vi "Set VI Icon.vi"(8 "error in (no error)":errorcluster, 10 "路径":path, 11 "VI引用句柄":refnum<vi>) -> (0 "error out":errorcluster, 1 "OK":bool, 2 "OldHandle":u32, 3 "ImageHandle":u32)   [LabVIEW 2019]
uses:
  user32.dll
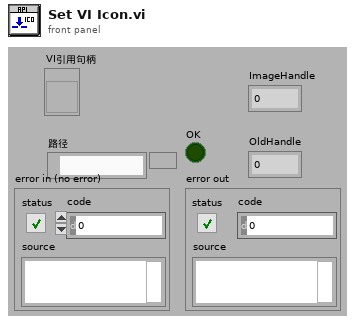
[diagram p1: front panel]
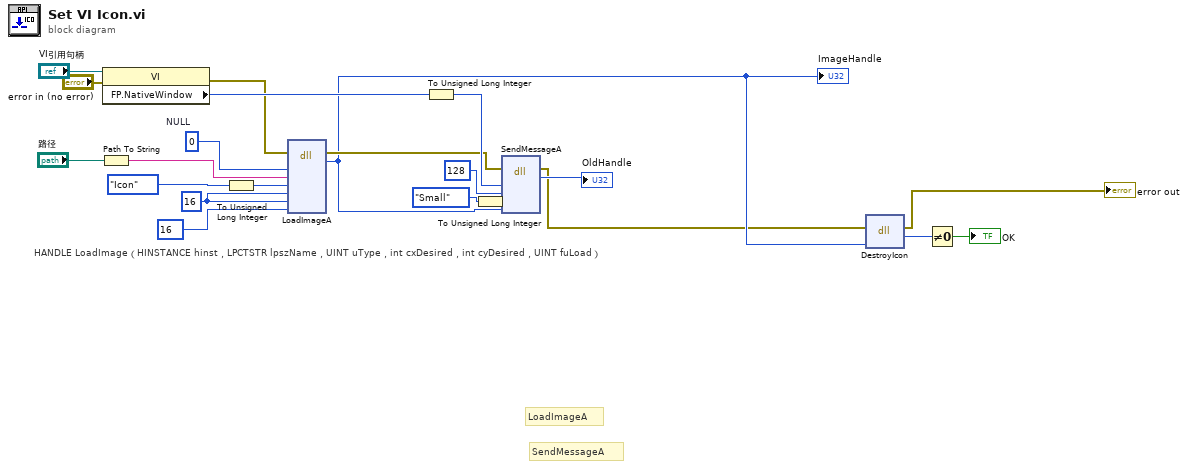
[diagram p0: block diagram]
diagram:
  w21 = u32 16 ("cxDesired")
  w22 = u32 0  # NULL
  # "SendMessageA"
  # "LoadImageA"
  # "HANDLE LoadImage（HINSTANCE hinst，LPCTSTR lpszName，UINT uType，int cxDesired，int cyDesired，UINT fuLoad）"
  n1 = Path To String(path="路径") -> (string=w19:string)
  n2 = property class="VI"(reference="VI引用句柄", error in="error in (no error)") -> (error out=w7:errorcluster, "FP.NativeWindow"=w13:u64)  [unwired: 1 out]
  n3 = To Unsigned Long Integer(number=enum32{"Bitmap", "Cursor", "Icon"}."Icon") -> (unsigned 32bit integer=w11:u32)
  n4 = dll-call lib="user32.dll" fn="LoadImageA" label="LoadImage"(error in=w7, "HINSTANCE"=w22, "LPCTSTR"=w19, "uType"=w11, "cxDesired"=w21, "cyDesired"=w21, "fuLoad"=16) -> (error out=w8:errorcluster, "ImageHandle"=w5:u32)  [unwired: 8 in, 1 out]
  "ImageHandle" <- w5
  n5 = To Unsigned Long Integer(number=w13) -> (unsigned 32bit integer=w10:u32)
  n6 = To Unsigned Long Integer(number=enum16{"Small", "Big"}."Small") -> (unsigned 32bit integer=w9:u32)
  n7 = dll-call lib="user32.dll" fn="SendMessageA" label="SendMessage"(error in=w8, "hWnd"=w10, "uMsg"=u32 128 ("dimension size"), "wParam"=w9, "lParam"=w5) -> (error out=w4:errorcluster, "OldHandle"=→"OldHandle":u32)  [unwired: 6 in, 1 out]
  n8 = dll-call lib="user32.dll" fn="DestroyIcon"(error in=w4, "hIcon"=w5) -> (error out=→"error out":errorcluster, "result"=w2:u32)  [unwired: 3 in, 1 out]
  n9 = Not Equal To 0?(x=w2) -> (x != 0?=→"OK":bool)
